vi "certaintyGraph With error.vi"() -> ()   [LabVIEW 2012]
panel:
  in  "Change":i16
  in  "Array":i16[][](array[numeric])
  in  "X":i16
  in  "Y":u16
  out "Array 2":i16[][](array[numeric])
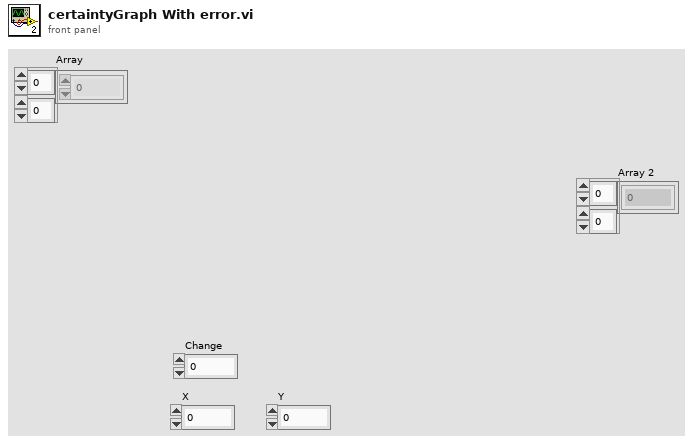
[diagram p1: front panel]
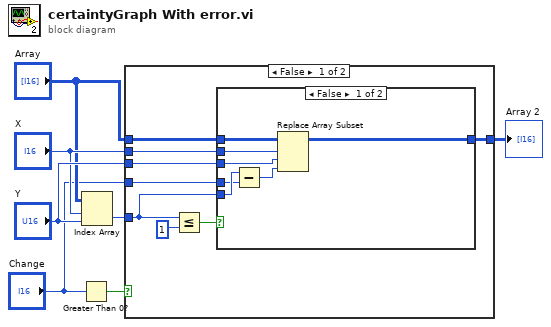
[diagram p0: block diagram]
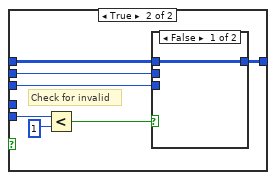
[diagram p2: hidden frame]
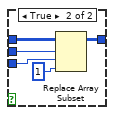
[diagram p3: hidden frame]
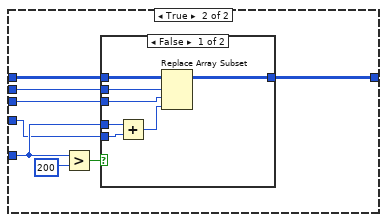
[diagram p4: hidden frame]
diagram:
  n1 = Greater Than 0?(x="Change") -> (x > 0?=w2:bool)
  n2 = Index Array(array="Array", index (row)="X", index (col)="Y") -> (element=w3:i16)
  n3 = case shown="False" w2 {
    tunnel: w3 -> [w13 w38]
    tunnel: "Array" -> [w12 w43]
    tunnel: "X" -> [w11 w42]
    tunnel: "Y" -> [w10 w41]
    tunnel: [w9 w37] -> w7
    tunnel: "Change" -> [w8 w36]
    frame False {
      n4 = Less Or Equal?(x=w13, y=1) -> (x <= y?=w14:bool)
      n5 = case shown="False" w14 {
        tunnel: w13 -> [w18 w29]
        tunnel: w12 -> [w22 w26]
        tunnel: w11 -> [w20 w25]
        tunnel: w10 -> [w19 w24]
        tunnel: [w21 w23] -> w9
        tunnel: w8 -> [w16 _]
        frame False {
          n6 = Subtract(x=w18, y=w16) -> (x-y=w17:i16)
          n7 = Replace Array Subset(array=w22, new element=w17, index (row)=w20, index (col)=w19) -> (w21:i16[][])
        }
        frame True {
          # "Check for invalid"
          n8 = Less?(x=w29, y=1) -> (x < y?=w27:bool)
          n9 = case shown="False" w27 {
            tunnel: w26 -> [w30 w35]
            tunnel: w25 -> [_ w34]
            tunnel: w24 -> [_ w33]
            tunnel: [w30 w31] -> w23
            frame False {
            }
            frame True {
              n10 = Replace Array Subset(array=w35, new element=1, index (row)=w34, index (col)=w33) -> (w31:i16[][])
            }
          }
        }
      }
    }
    frame True {
      n11 = Greater?(x=w38, y=200) -> (0:w39:bool)
      n12 = case shown="False" w39 {
        tunnel: w43 -> [w46 w51]
        tunnel: w42 -> [w50 _]
        tunnel: w41 -> [w49 _]
        tunnel: w38 -> [w48 _]
        tunnel: [w45 w51] -> w37
        tunnel: w36 -> [w44 _]
        frame False {
          n13 = Add(x=w48, y=w44) -> (x+y=w47:i16)
          n14 = Replace Array Subset(array=w46, new element=w47, index (row)=w50, index (col)=w49) -> (w45:i16[][])
        }
        frame True {
          # "Certainty cant go higher"
        }
      }
    }
  }
  "Array 2" <- w7
